vi "Trigger Maker from TTL Input.vi"(6 "Trigger Delay Alazar":u32=150, 8 "Error in":errorcluster, 11 "Master Trigger In from Laser (TTL)":tag="/Dev1/PFI7") -> (0 "error out":errorcluster, 2 "Alazar Task":refnum<k21>, 3 "AFG11000 Task":refnum<k21>)   [LabVIEW 2014]
uses:
  <vilib>/DAQmx/create/channels.llb/DAQmx Create Channel (CO-Pulse Generation-Ticks).vi
  <vilib>/DAQmx/configure/trigger.llb/DAQmx Start Trigger (Digital Edge).vi
  <resource>/objmgr/daqmx.rc
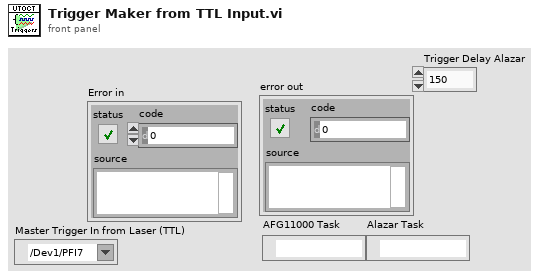
[diagram p1: front panel]
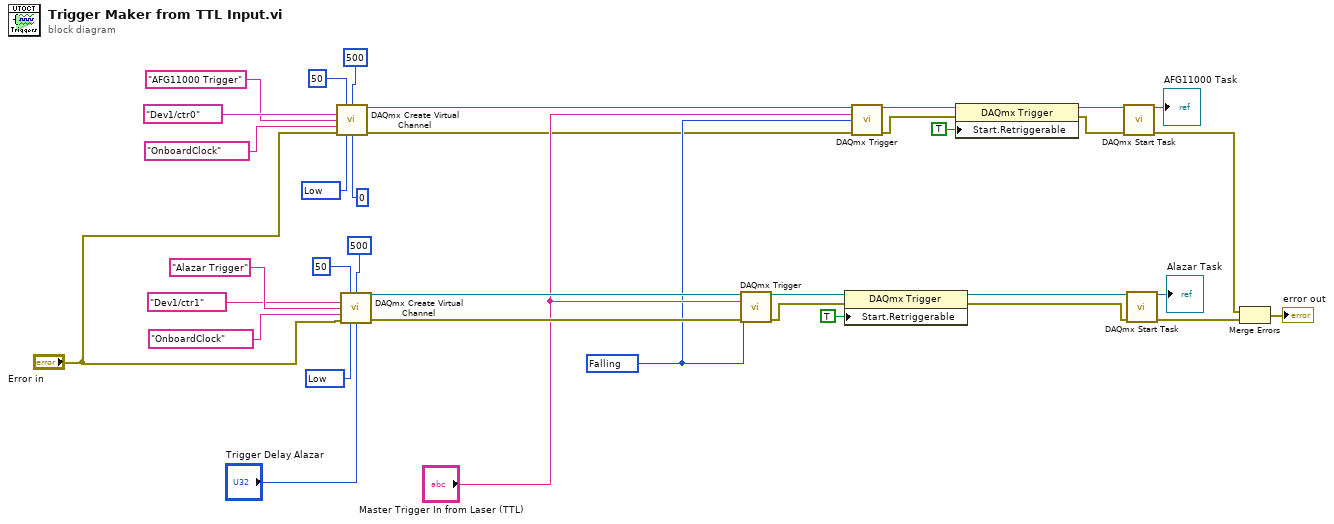
[diagram p0: block diagram]
diagram:
  w2 = 10171 items=["Rising"=10280, "Falling"=10171] ("edge")
  w18 = 10214 items=["High"=10192, "Low"=10214] ("idle state")
  w35 = 10214 items=["High"=10192, "Low"=10214] ("idle state")
  n1 = call-poly <vilib>:"DAQmx Create Virtual Channel.vi"("high ticks"=u32 50, "low ticks"=u32 500, "counter"=tag "Dev1/ctr0", "name to assign"="AFG11000 Trigger", "source of ticks"=tag "OnboardClock", "error in"="Error in", "idle state"=w35, "initial delay"=u32 0) -> ("task out"=w24:refnum<k21>, "error out"=w1:errorcluster)  [unwired: 6 in]
  n2 = call-poly <vilib>:"DAQmx Create Virtual Channel.vi"("high ticks"=u32 50, "low ticks"=u32 500, "counter"=tag "Dev1/ctr1", "name to assign"="Alazar Trigger", "source of ticks"=tag "OnboardClock", "error in"="Error in", "idle state"=w18, "initial delay"="Trigger Delay Alazar") -> ("task out"=w12:refnum<k21>, "error out"=w13:errorcluster)  [unwired: 6 in]
  n3 = call-poly <vilib>:"DAQmx Trigger.vi"("task/channels in"=w12, "source"="Master Trigger In from Laser (TTL)", "edge"=w2, "error in"=w13) -> ("task out"=w14:refnum<k21>, "error out"=w16:errorcluster)  [unwired: 10 in]
  n4 = property class="DAQmx Trigger"(reference=w14, error in=w16, "Start.Retriggerable"=TRUE) -> (reference out=w11:refnum<k21>, error out=w10:errorcluster)
  n5 = call-poly <vilib>:"DAQmx Trigger.vi"("task/channels in"=w24, "source"="Master Trigger In from Laser (TTL)", "edge"=w2, "error in"=w1) -> ("task out"=w29:refnum<k21>, "error out"=w26:errorcluster)  [unwired: 10 in]
  n6 = property class="DAQmx Trigger"(reference=w29, error in=w26, "Start.Retriggerable"=TRUE) -> (reference out=w27:refnum<k21>, error out=w25:errorcluster)
  n7 = call <vilib>:"DAQmx Start Task.vi"("task/channels in"=w27, "error in"=w25) -> ("task out"=→"AFG11000 Task":refnum<k21>, "error out"=w8:errorcluster)  [unwired: 12 in]
  n8 = call <vilib>:"DAQmx Start Task.vi"("task/channels in"=w11, "error in"=w10) -> ("task out"=→"Alazar Task":refnum<k21>, "error out"=w9:errorcluster)  [unwired: 12 in]
  n9 = Merge Errors(w8, w9) -> (→"error out":errorcluster)
